vi "ChildImplementationDefaultValue--Constant.vi"() -> (3 "ChildImplementationDefaultValue":string)   [LabVIEW 2021, in "lv_icon.lvlib"]
uses:
  <vilib>/LabVIEW Icon API/lv_icon/lv_icon.lvlib
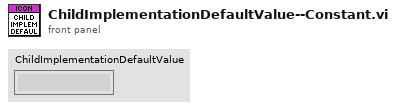
[diagram p1: front panel]
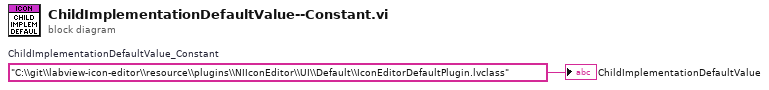
[diagram p0: block diagram]
diagram:
  w1 = "C:\\git\\labview-icon-editor\\resource\\plugins\\NIIconEditor\\UI\\Default\\IconEditorDefaultPlugin.lvclass"  # ChildImplementationDefaultValue_Constant
  "ChildImplementationDefaultValue" <- w1
